vi "DB_CargaEquipos.vi"(8 "error in (no error)":errorcluster, 11 "db in":T1) -> (0 "error out":errorcluster, 1 "Equipos":string[][](array[string]), 2 "Equipos_out":T2[](array[typedef]), 3 "db out":T1, 4 "NOMBRE_EQUIPOS":string[](array[string]), 5 "ID_EQUIPOS":i32[](array[numeric]), 6 "ESTADO_EQUIPO":string[](array[string]), 7 "IP_EQUIPOS":string[](array[string]))   [LabVIEW 2018]
uses:
  Controls/Equipos_Medicion_cluster.ctl
  <vilib>/addons/database/Connection.llb/Conn ObjectReference.ctl
  <vilib>/Utility/sysdir.llb/System Directory Type.ctl
  <vilib>/Utility/file.llb/Read Delimited Spreadsheet (string).vi
  <vilib>/addons/database/Connection.llb/Conn Execute.vi
  <vilib>/addons/database/Recordset.llb/Rec Fetch Recordset Data (R).vi
  <vilib>/addons/database/Recordset.llb/Rec Destroy - Connection.vi
  <vilib>/addons/database/_DB Variant To Data/Database Variant To Data.xnode
  <vilib>/addons/database/NI_Database_API.lvlib
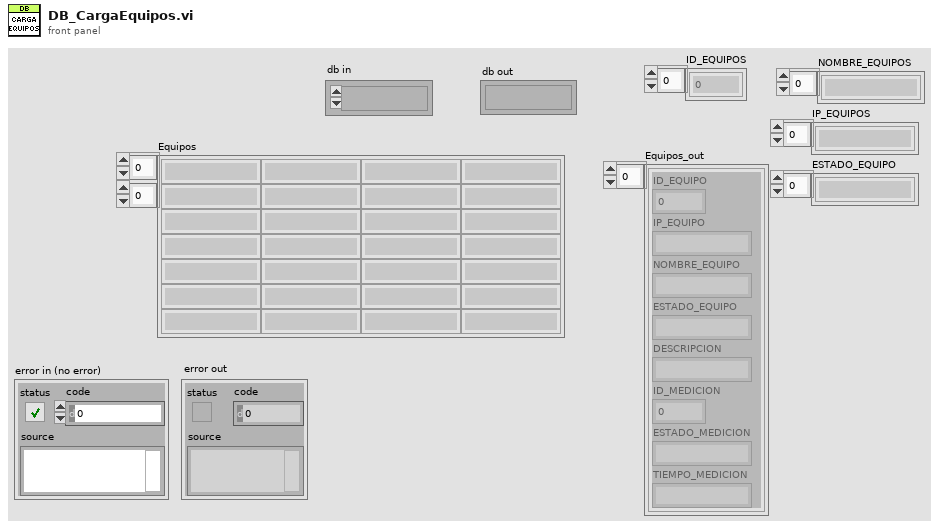
[diagram p1: front panel]
types:
  T1 = typedef "NI_Database_API.lvlib/Conn ObjectReference.ctl" = refnum<k1>
  T2 = typedef "Equipos_Medicion_cluster.ctl" = cluster{"ID_EQUIPO":i32, "IP_EQUIPO":string, "NOMBRE_EQUIPO":string, "ESTADO_EQUIPO":string, "DESCRIPCION":string, "ID_MEDICION":i32, "ESTADO_MEDICION":string, "TIEMPO_MEDICION":string}
  T3 = typedef "System Directory Type.ctl" = i32
  T4 = typedef "NI_Database_API.lvlib/Rec ObjectReference.ctl" = refnum<k1>
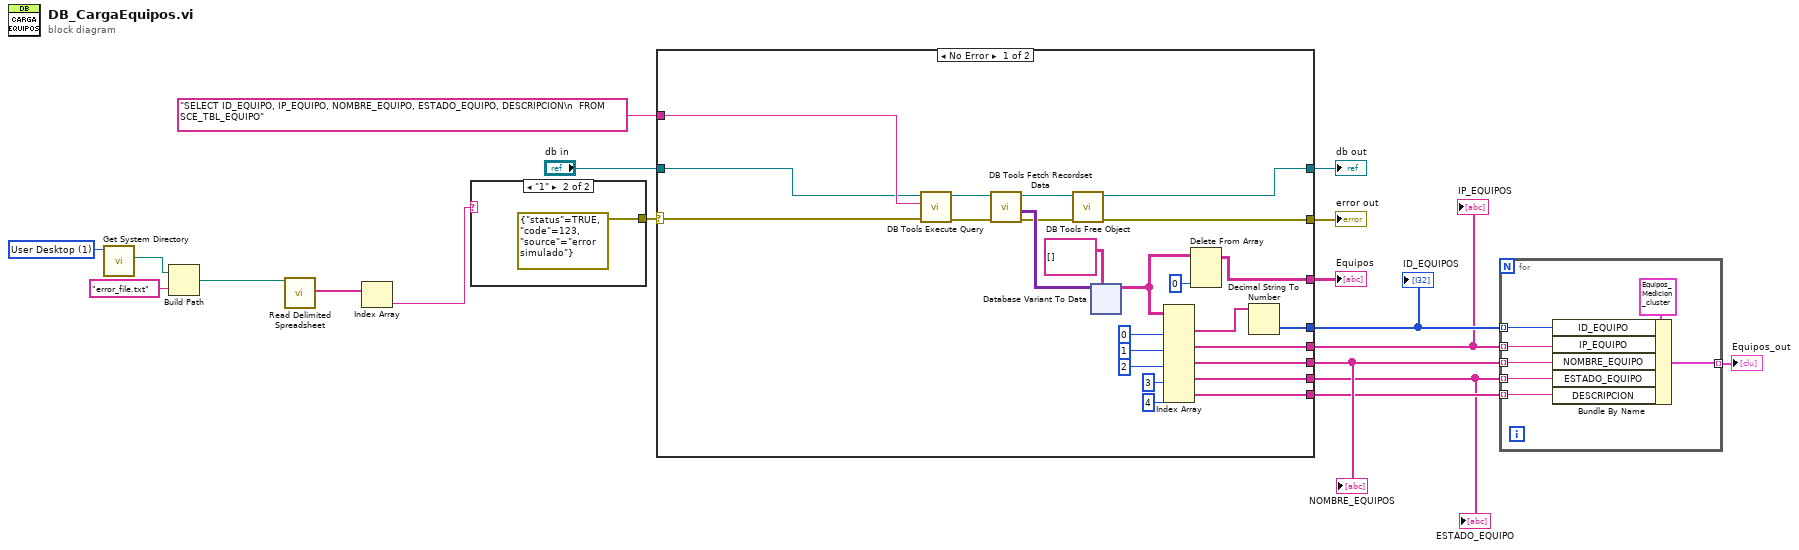
[diagram p0: block diagram]
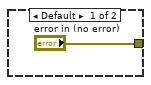
[diagram p2: hidden frame]
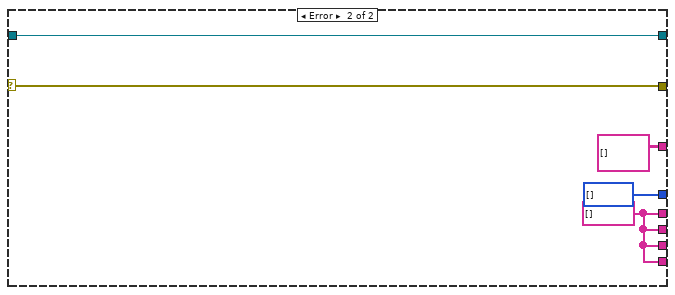
[diagram p3: hidden frame]
diagram:
  w6 = T3 1 items=["User Home"=0, "User Desktop"=1, "User Documents"=2, "User Application Data"=3, "User Preferences"=4, "User Temporary"=5, "Public Documents"=6, "Public Application Data"=7, "Public Preferences"=8, "Public Cache"=13, "System Core Libraries"=9, "System Installed Libraries"=10, "Application Files"=11, "Boot Volume Root"=12] ("system directory type")
  n1 = call <vilib>:"Get System Directory.vi"("system directory type"=w6) -> ("system directory"=w5:path)  [unwired: 10 in]
  n2 = Build Path(base path=w5, name or relative path="error_file.txt") -> (appended path=w3:path)
  n3 = call-poly <vilib>:"Read Delimited Spreadsheet.vi"("file path (dialog if empty)"=w3) -> ("first row"=w2:string[])  [unwired: 9 in, 5 out]
  n4 = Index Array(array=w2) -> (element=w1:string)  [unwired: 1 in]
  n5 = case shown="\"1\"" w1 {
    tunnel: ["error in (no error)" errorcluster {"status"=TRUE, "code"=123, "source"="error simulado"} ("error in (error)")] -> w17
    frame Default {
    }
    frame "1" {
    }
  }
  n6 = case shown="No Error" w17 {
    selector: w17 -> [w43 w94]
    tunnel: [w45 w94] -> w18
    tunnel: "SELECT ID_EQUIPO, IP_EQUIPO, NOMBRE_EQUIPO, ESTADO_EQUIPO, DESCRIPCION\n  FROM SCE_TBL_EQUIPO" ("SQL") -> [w42 _]
    tunnel: [w35 i32[] []] -> w15
    tunnel: [w34 w92] -> w14
    tunnel: [w33 w92] -> w13
    tunnel: [w32 w92] -> w12
    tunnel: [w26 w92] -> w10
    tunnel: [w23 string[][] [] ("data")] -> w9
    tunnel: "db in" -> [w22 w90]
    tunnel: [w21 w90] -> w7
    frame No Error {
      n7 = call-poly <vilib>:"DB Tools Execute Query.vi"("error in (no error)"=w43, "SQL query"=w42, "connection reference"=w22) -> ("error out"=w44:errorcluster, "recordset reference"=w41:T4)  [unwired: 5 in]
      n8 = call-poly <vilib>:"DB Tools Fetch Recordset Data.vi"("error in (no error)"=w44, "recordset reference"=w41) -> ("error out"=w37:errorcluster, "recordset data"=w38:variant[][], "recordset reference out"=w40:T4)  [unwired: 3 in]
      n9 = call-poly <vilib>:"DB Tools Free Object.vi"("error in (no error)"=w37, "recordset reference"=w40) -> ("error out"=w45:errorcluster, "connection reference"=w21:T1)  [unwired: 8 in]
      n10 = xnode "Database Variant To Data"("database variant"=w38, "type"=string[][] []) -> ("data"=w25:string[][])  [unwired: 1 in, 1 out]
      n11 = Index Array(array=w25, index (col) #1=0 ("disabled index (col)"), index (col) #2=1 ("index (col)"), index (col) #3=2 ("index (col)"), index (col) #4=3 ("index (col)"), index (col) #5=4 ("index (col)")) -> (element #1=w36:string[], element #2=w34:string[], element #3=w33:string[], element #4=w26:string[], element #5=w32:string[])  [unwired: 5 in]
      n12 = Delete From Array(array=w25, index (col)=0 ("disabled index (col)")) -> (array with subset deleted=w23:string[][])  [unwired: 2 in, 1 out]
      n13 = Decimal String To Number(string=w36) -> (number=w35:i32[])  [unwired: 2 in, 1 out]
    }
    frame Error {
      w92 = string[] [] ("data")
    }
  }
  "error out" <- w18
  "Equipos" <- w9
  "db out" <- w7
  "ID_EQUIPOS" <- w15
  "NOMBRE_EQUIPOS" <- w13
  "IP_EQUIPOS" <- w14
  "ESTADO_EQUIPO" <- w10
  n14 = for {
    tunnel: w15 -> [w100] mode=indexing
    tunnel: w14 -> [w99] mode=indexing
    tunnel: w13 -> [w98] mode=indexing
    tunnel: w12 -> [w95] mode=indexing
    tunnel: [w97] -> w11 mode=indexing
    tunnel: w10 -> [w96] mode=indexing
    n15 = Bundle By Name(cluster=T2 {"ID_EQUIPO"=0, "IP_EQUIPO"="", "NOMBRE_EQUIPO"="", "ESTADO_EQUIPO"="", "DESCRIPCION"="", "ID_MEDICION"=0, "ESTADO_MEDICION"="", "TIEMPO_MEDICION"="12-02-2019 18:41"} ("Equipo_Medicion"), "ID_EQUIPO"=w100, "IP_EQUIPO"=w99, "NOMBRE_EQUIPO"=w98, "ESTADO_EQUIPO"=w96, "DESCRIPCION"=w95) -> (w97:T2)
  }
  "Equipos_out" <- w11
